vi "timestamp_to_postgres_date.vi"(8 "error in (no error)":errorcluster, 10 "utc":bool, 11 "date_time":dbl format="%^<%H:%M:%S%4u %m/%d/%y>T") -> (0 "error out":errorcluster, 3 "postgres_date":string)   [LabVIEW 2015, in "lv-timescaledb.lvlib"]
uses:
  lv-timescaledb.lvlib
  <vilib>/addons/database/NI_Database_API.lvlib
  <vilib>/addons/database/Auxilliary.llb/DB Tools Format Datetime String (Time Stamp).vi
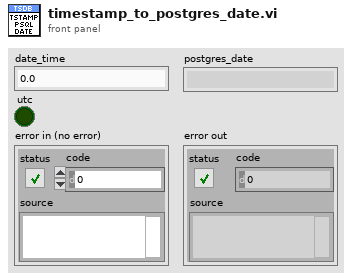
[diagram p1: front panel]
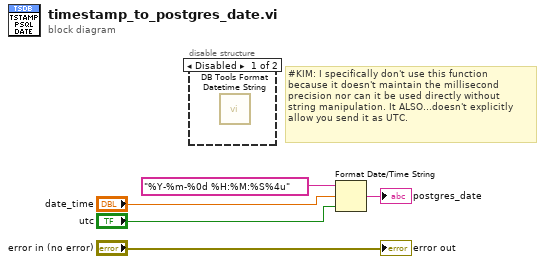
[diagram p0: block diagram]
diagram:
  # "#KIM: I specifically don't use this function\nbecause it doesn't maintain the millisecond\nprecision nor can it be used directly without\nstring manipulation. It ALSO...doesn't explicitly\nallow you send it as UTC."
  n1 = disable-structure shown="Disabled" {
    frame Disabled {
      n2 = call-poly <vilib>:"DB Tools Format Datetime String.vi"() -> ()  [unwired: 1 in, 1 out]
    }
    frame Enabled {
    }
  }
  n3 = Format Date/Time String(time format string (%c)="%Y-%m-%0d %H:%M:%S%4u", seconds (now)="date_time", UTC format="utc") -> (date/time string=→"postgres_date":string)
  "error out" <- "error in (no error)"
